vi "Read D-Register.vi"(8 "error in":errorcluster, 10 "D-register number":u32=1, 11 "VISA resource name":refnum<visa-resource-name>) -> (0 "error out":errorcluster, 2 "Data":u32, 3 "VISA resource name out":refnum<visa-resource-name>, 5 "Data Valid":bool)   [LabVIEW 2017, in "Samwontech TEMP2xxx.lvlib"]
uses:
  <instrlib>/Samwontech TEMP2xxx/Samwontech TEMP2xxx.lvlib
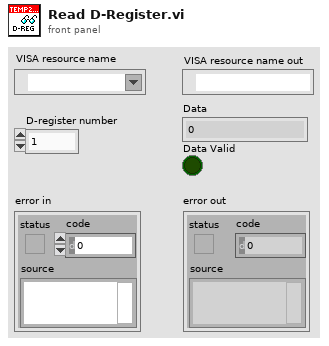
[diagram p1: front panel]
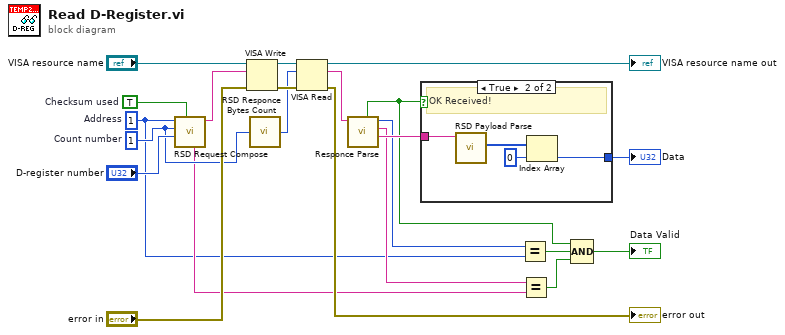
[diagram p0: block diagram]
diagram:
  w13 = u8 1  # Count number
  w5 = u8 1  # Address
  w22 = TRUE  # Checksum used
  n1 = call <instrlib>:"RSD Request Compose.vi"("Checksum used"=w22, "D-register number"="D-register number", "Count number"=w13, "Address"=w5) -> ("Request"=w19:string, "Command"=w7:string)  [unwired: 6 in]
  n2 = VISA Write(VISA resource name="VISA resource name", write buffer=w19, error in (no error)="error in") -> (VISA resource name out=w17:refnum<visa-resource-name>, error out=w14:errorcluster)  [unwired: 1 out]
  n3 = call <instrlib>:"RSD Responce Bytes Count.vi"("Count Number"=w13) -> ("Bytes Count"=w12:u32)
  n4 = VISA Read(VISA resource name=w17, byte count=w12, error in (no error)=w14) -> (VISA resource name out=→"VISA resource name out":refnum<visa-resource-name>, read buffer=w11:string, error out=→"error out":errorcluster)  [unwired: 1 out]
  n5 = call <instrlib>:"Responce Parse.vi"("Responce"=w11) -> ("Payload"=w9:string, "Command"=w8:string, "Address"=w6:u8, "OK"=w2:bool)  [unwired: 6 in, 1 out]
  n6 = case shown="True" w2 {
    tunnel: [_ w23] -> w10
    tunnel: w9 -> [_ w24]
    frame False {
    }
    frame True {
      # "OK Received!"
      n7 = call <instrlib>:"RSD Payload Parse.vi"("Payload"=w24) -> ("Data (number)"=w26:u32[])  [unwired: 9 in, 1 out]
      n8 = Index Array(array=w26, index=0) -> (element=w23:u32)
    }
  }
  "Data" <- w10
  n9 = Equal?(x=w6, y=w5) -> (x = y?=w3:bool)
  n10 = Equal?(x=w8, y=w7) -> (x = y?=w4:bool)
  n11 = Compound Arithmetic op=AND(w2, w3, w4) -> (→"Data Valid":bool)
